vi "SCT Get FP Paths.vi"(1 "localized names":string[](array[string]), 2 "internal names":string[](array[string])) -> (0 "Array":path[](array[path]))   [LabVIEW 2016]
uses:
  <vilib>/Utility/error.llb/DialogType.ctl
  <resource>/dialog/variable/SCT Localization Strings.vi
  <vilib>/variable/NI_Variable.lvlib
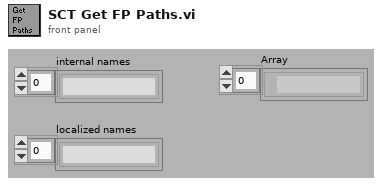
[diagram p1: front panel]
types:
  T1 = typedef "DialogType.ctl" = u16
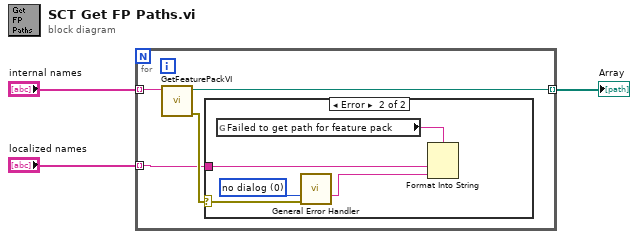
[diagram p0: block diagram]
diagram:
  n1 = for {
    tunnel: "internal names" -> [w7] mode=indexing
    tunnel: [w6] -> w2 mode=indexing
    tunnel: "localized names" -> [w4] mode=indexing
    n2 = call <vilib>:"GetFeaturePackVI.vi"("fpName"=w7) -> ("error out"=w5:errorcluster, "path"=w6:path)  [unwired: 9 in]
    n3 = case shown="Error" w5 {
      selector: w5 -> [_ w10]
      tunnel: w4 -> [_ w11]
      frame No Error {
      }
      frame Error {
        w9 = T1 0 items=["no dialog", "OK message", "continue or stop message", "OK message + warnings", "continue/stop + warnings"] ("type of dialog (OK msg:1)")
        n4 = global read "SCT Localization Strings.vi" "Failed to get path for feature pack"() -> (w12:string)
        n5 = call <vilib>:"General Error Handler.vi"("type of dialog (OK msg:1)"=w9, "error in (no error)"=w10) -> ("message"=w8:string)  [unwired: 9 in, 4 out]
        n6 = Format Into String(format string=w12, w11, w8) -> ()  [unwired: 2 in, 2 out]
      }
    }
  }
  "Array" <- w2
